vi "Connect.vi"(8 "error in":errorcluster, 11 "Modbus in":refnum<class "Modbus.lvclass">) -> (0 "error out":errorcluster, 3 "Modbus out":refnum<class "Modbus.lvclass">)   [LabVIEW 2021, in "Modbus.lvclass"]
uses:
  Modbus.lvclass
  controls/INI FGV States.ctl
  Modbus.lvclass/Modbus.ctl
  <vilib>/NI/Modbus Library/API/Wrapper/Create TCP Master.vi
  <vilib>/NI/Modbus Library/API/Wrapper/API Main.lvlib
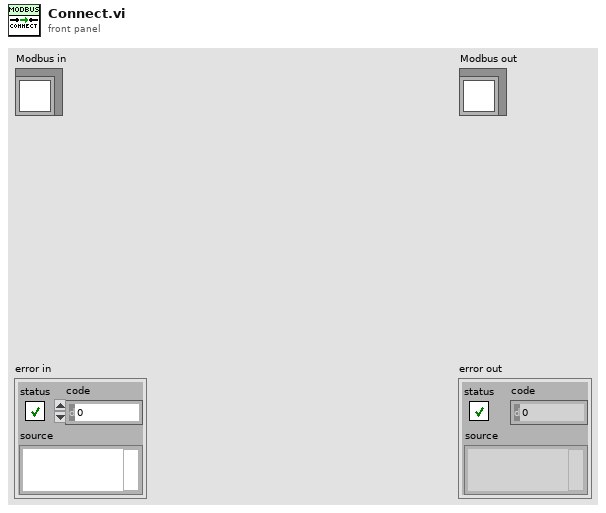
[diagram p1: front panel]
types:
  T1 = typedef "INI FGV States.ctl" = enum16{"Open File", "Read Config", "Write Config", "Close File"}
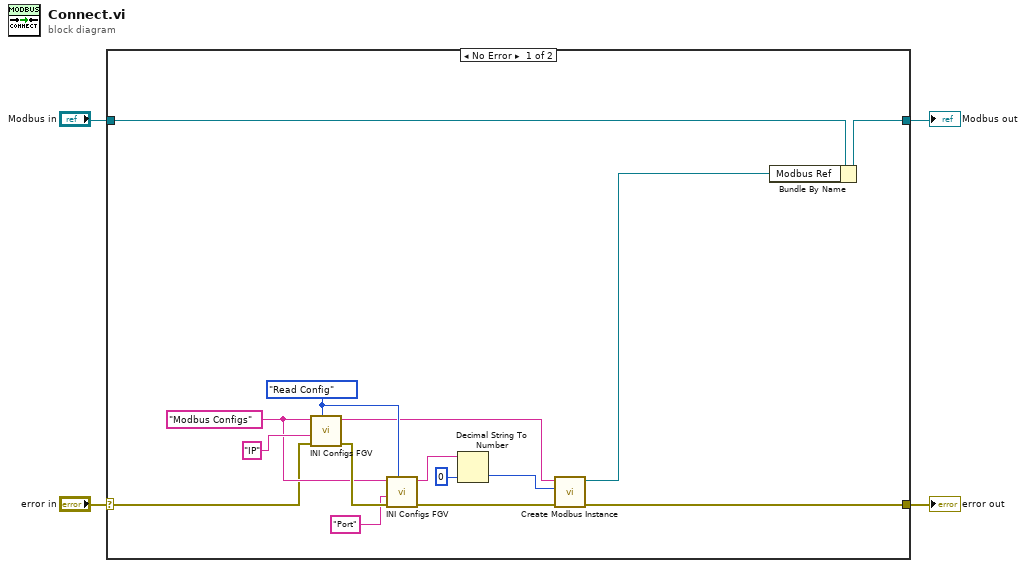
[diagram p0: block diagram]
diagram:
  n1 = case shown="No Error" "error in" {
    selector: "error in" -> [w10 w20]
    tunnel: [w18 w20] -> w3
    tunnel: [w6 w21] -> w2
    tunnel: "Modbus in" -> [w19 w21]
    frame No Error {
      w15 = "Modbus Configs" ("section")
      w13 = INI_FGV_States."Read Config" ("State")
      n2 = call "INI Configs FGV.vi"("State"=w13, "error in"=w10, "key"="IP", "section"=w15) -> ("error out"=w16:errorcluster, "value"=w8:string)  [unwired: 6 in]
      n3 = call "INI Configs FGV.vi"("State"=w13, "error in"=w16, "key"="Port", "section"=w15) -> ("error out"=w9:errorcluster, "value"=w12:string)  [unwired: 6 in]
      n4 = Decimal String To Number(string=w12, default (0L)=u16 0 ("remote port or service name")) -> (number=w7:u16)  [unwired: 1 in, 1 out]
      n5 = call-poly <vilib>:"Create Modbus Instance.vi"("error in"=w9, "port (502)"=w7, "address"=w8) -> ("error out"=w18:errorcluster, "TCP master instance"=w5:refnum<class "Modbus Master.lvclass">)  [unwired: 7 in]
      n6 = Bundle By Name(cluster=w19, "Modbus Ref"=w5) -> (w6:refnum<class "Modbus.lvclass">)
    }
    frame Error {
    }
  }
  "error out" <- w3
  "Modbus out" <- w2
